vi "Data Viewer.vi"() -> ()   [LabVIEW 2014]
uses:
  TypeDef/Q1 Viewer.ctl
panel:
  out "ini file path":path
  out "Waveform Graph":waveform(dbl)[](graph)
  in  "Mode Selector":cluster{"Online Viewer":bool, "Navigator":bool}
  out "State":u16(ring) items=["initialize", "idle", "navigator", "online viewer", "exit"]
  in  "initialize":bool
  in  "referesh":bool
  in  "Cycle Time":i64=100 min=-1 step=1 format="%.0f msec"
  out "Sampling Interval":dbl min=0.0 step=1.0 format="%#_g msec"
  in  "Length (samples)":i64=1000 min=-1 step=1
  out "chart":waveform(dbl)[](graph)
  out "Start at sample":i32 min=0 step=1
  in  "Scrollbar":i32(c297)
  out "Number of Data":dbl format="%#_6f"
  in  "Variables":i32[](listbox)
  in  "Group Names":i32(listbox)
  in  "File Path Control":path caption="Open TDMS file:"
  out "Date":string
  out "Time":string
  in  "Stop Button":bool
  # "Data Viewer"
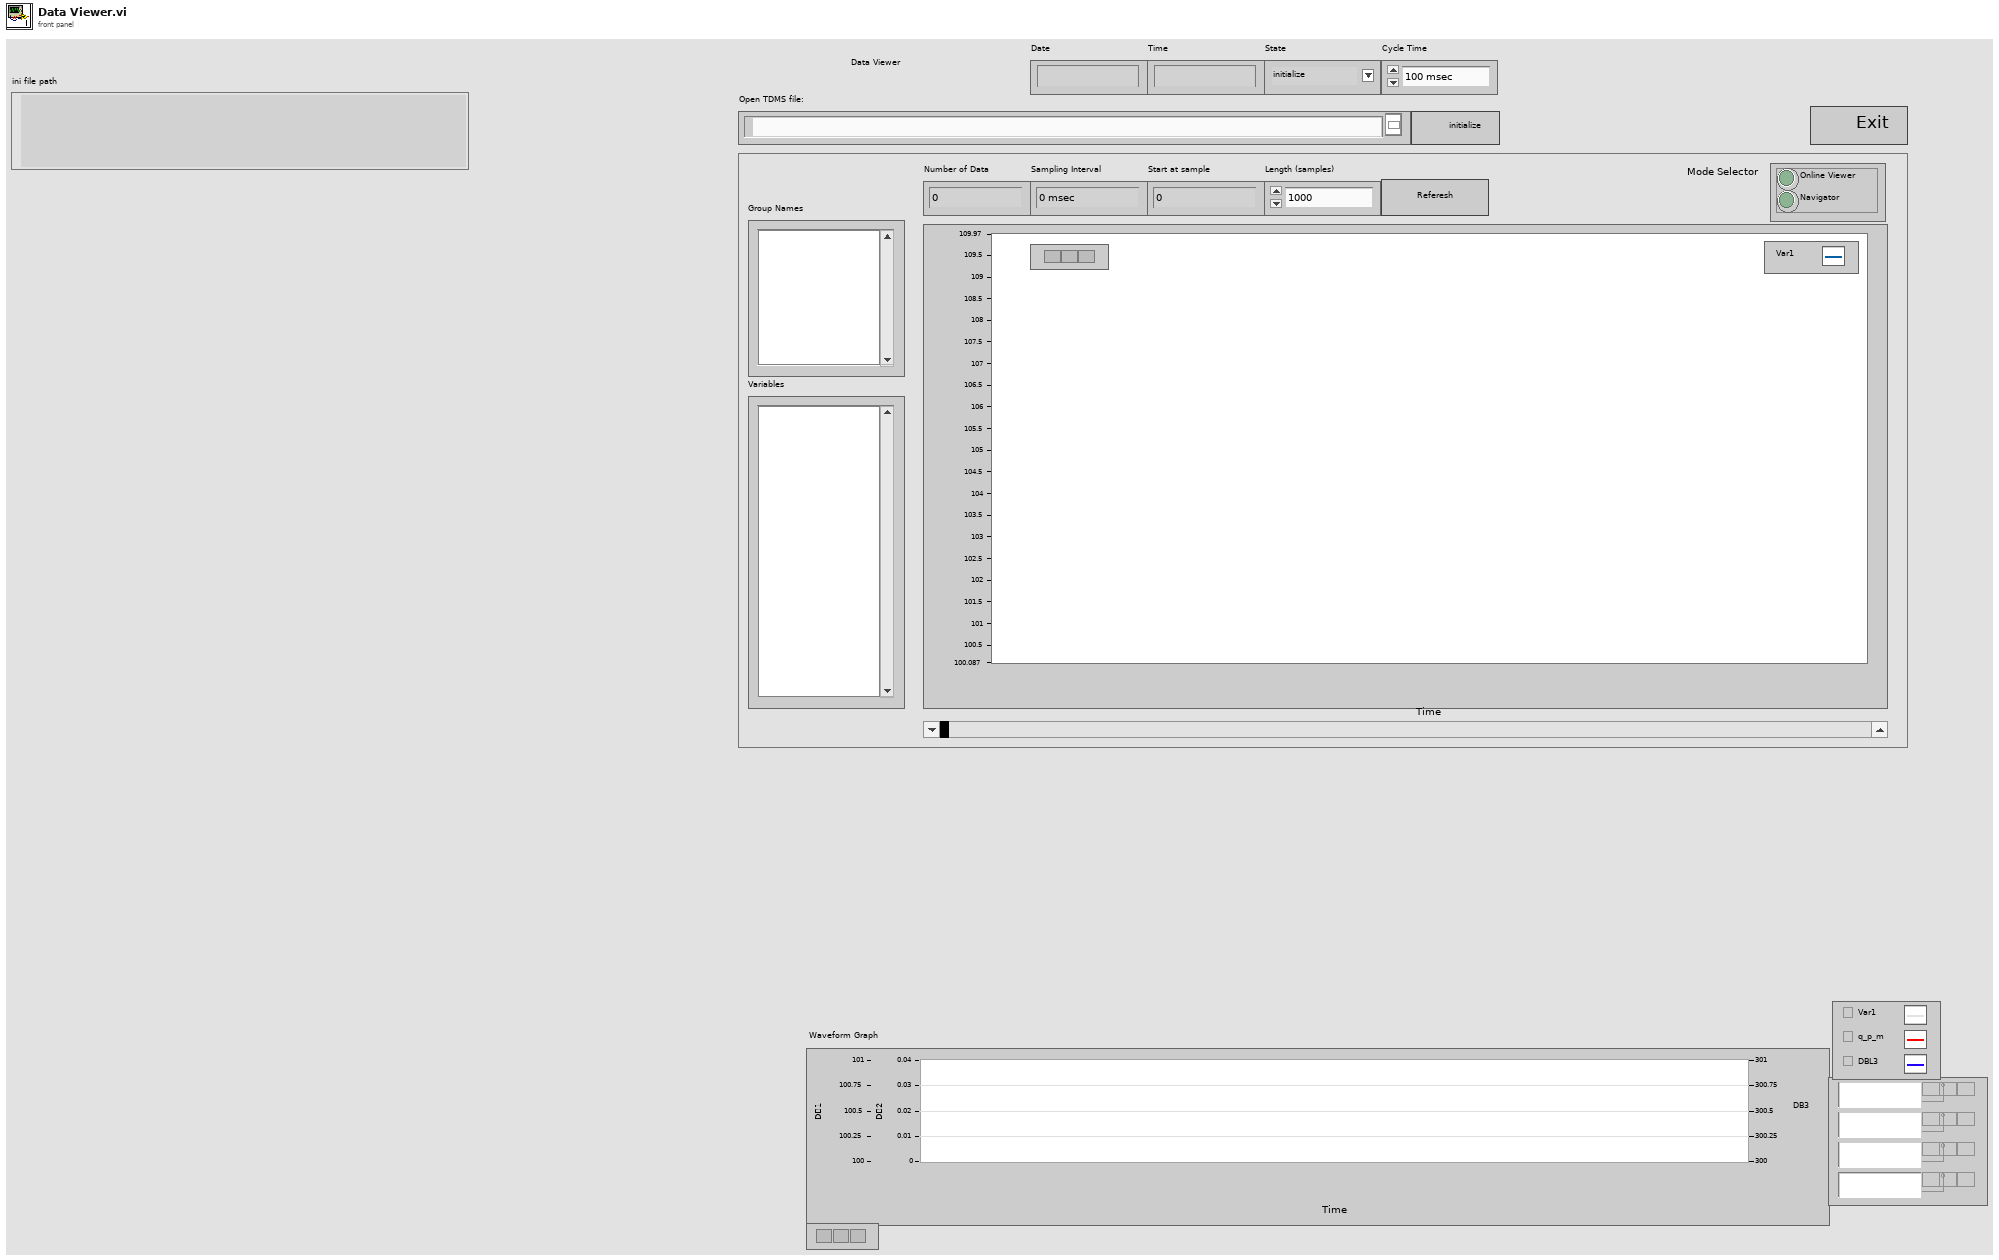
[diagram p1: front panel]
types:
  T1 = cluster{"Folder Path containing version information":path, "File name (including .ini)":path, "Section":string}
  T2 = typedef "Q1 Viewer.ctl" = cluster{"state":enum16{"initialize", "idle", "navigator", "online viewer", "exit"}, "data":variant}
  T3 = cluster{"path":path, "This VI":refnum<vi>, "Level of Application":u8}
  T4 = enum16{"open", "open or create", "create or replace", "create", "open (read-only)"}
  T5 = enum16{"initialize", "idle", "navigator", "online viewer", "exit"}
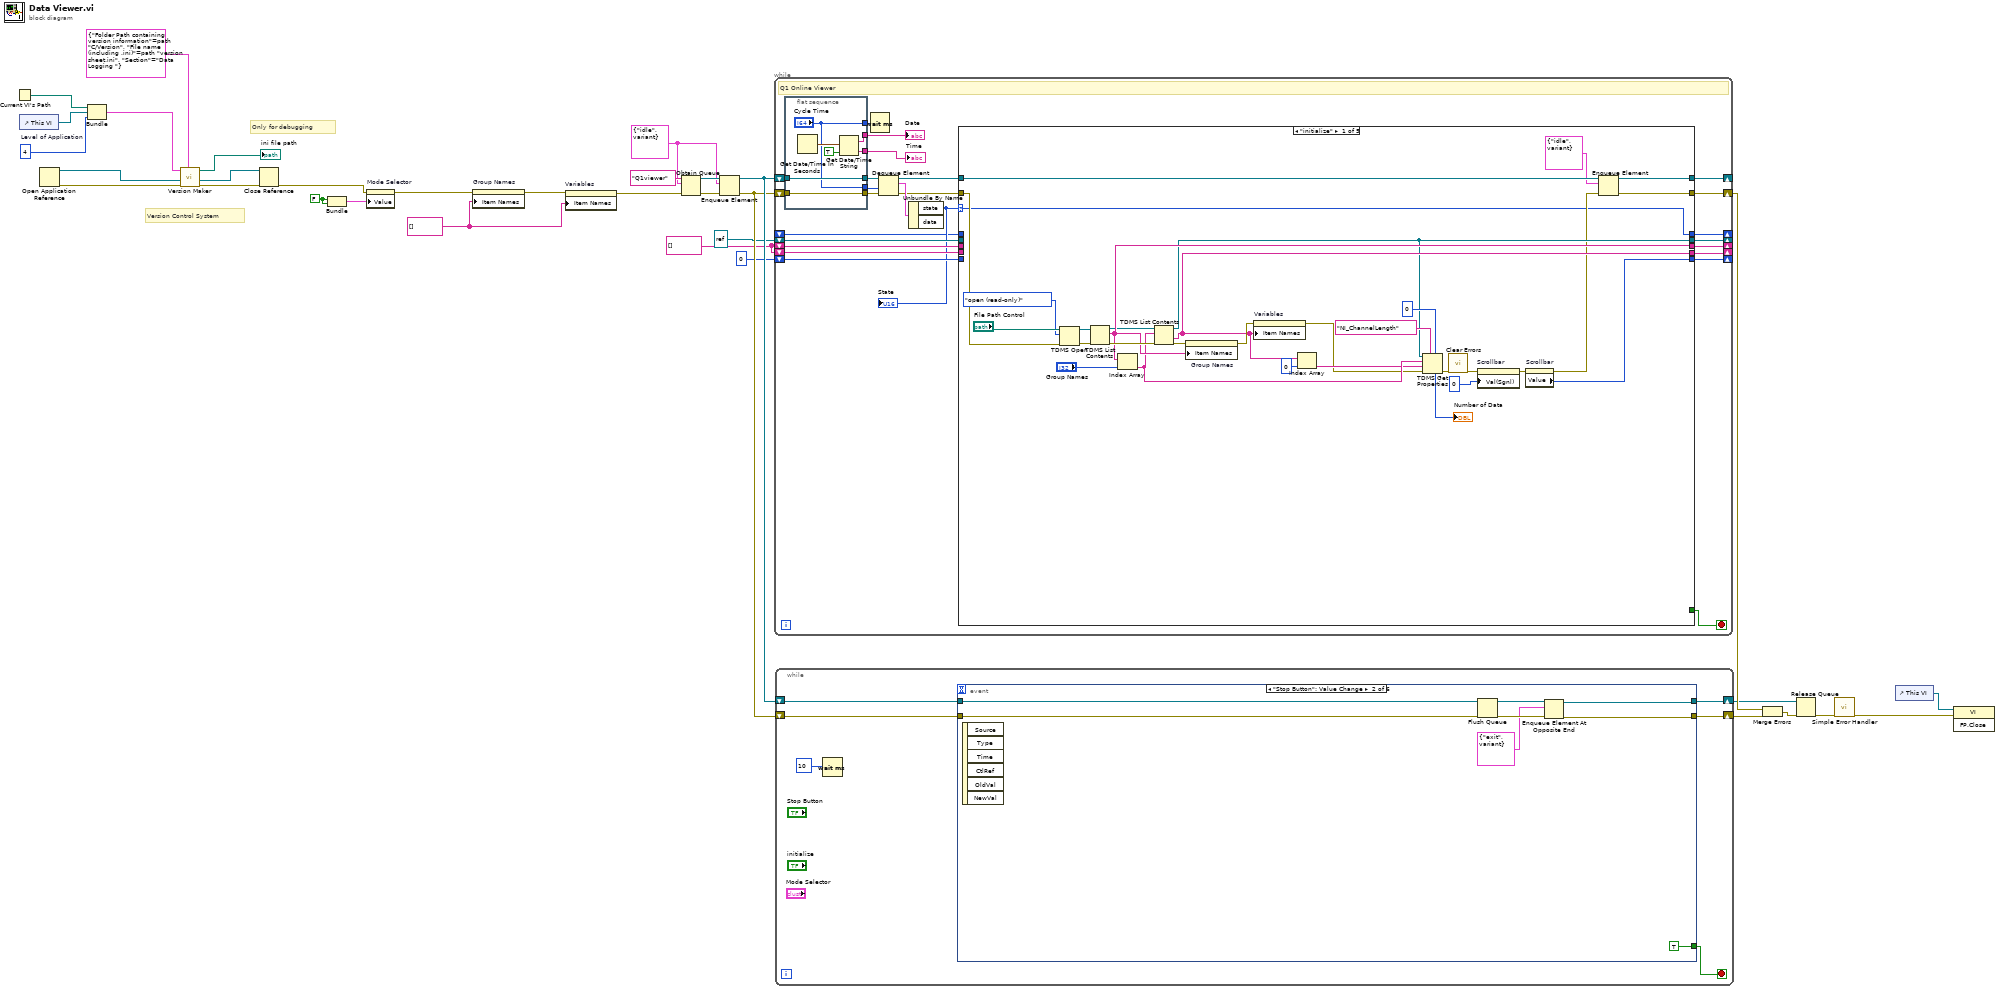
[diagram p0: block diagram]
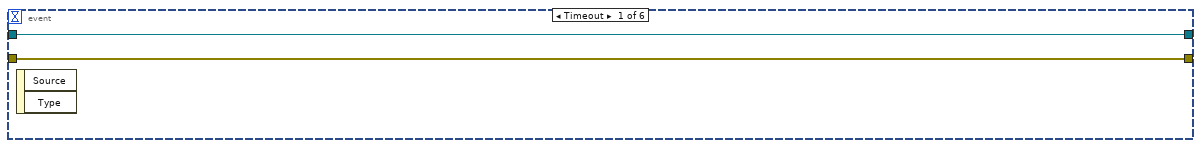
[diagram p2: hidden frame]
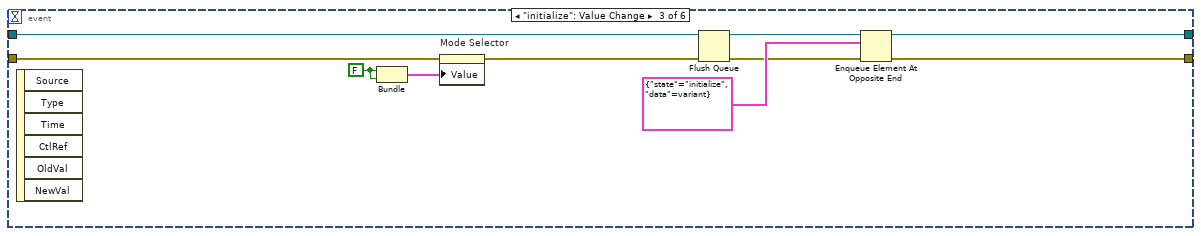
[diagram p3: hidden frame]
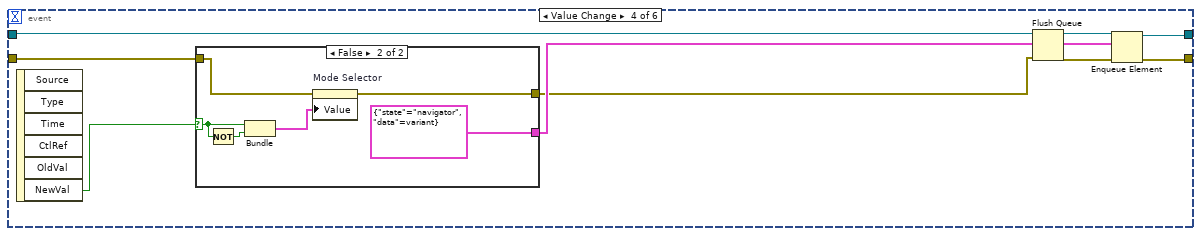
[diagram p4: hidden frame]
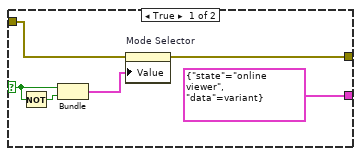
[diagram p5: hidden frame]
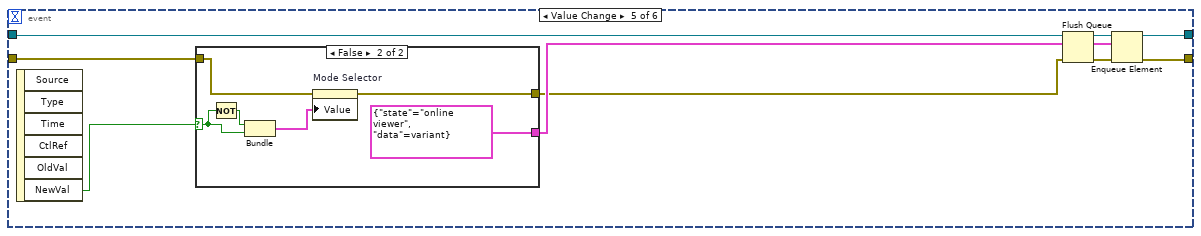
[diagram p6: hidden frame]
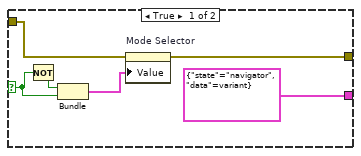
[diagram p7: hidden frame]
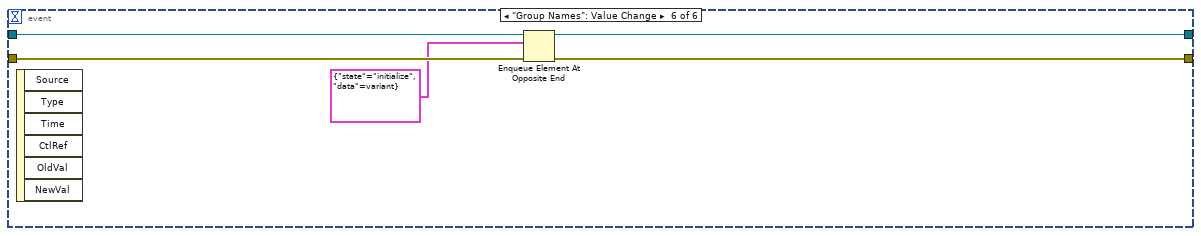
[diagram p8: hidden frame]
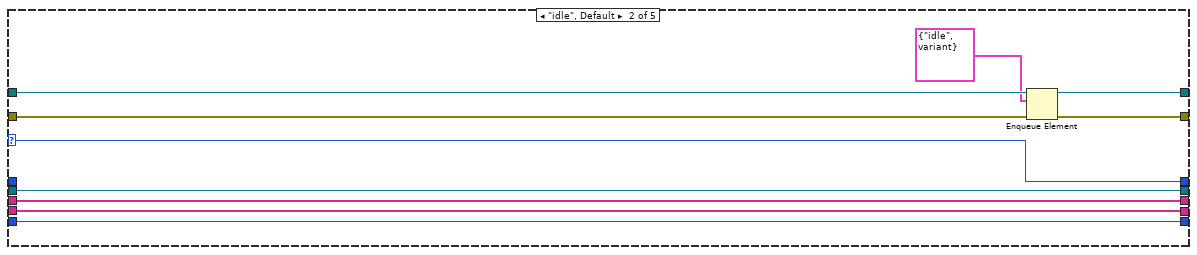
[diagram p9: hidden frame]
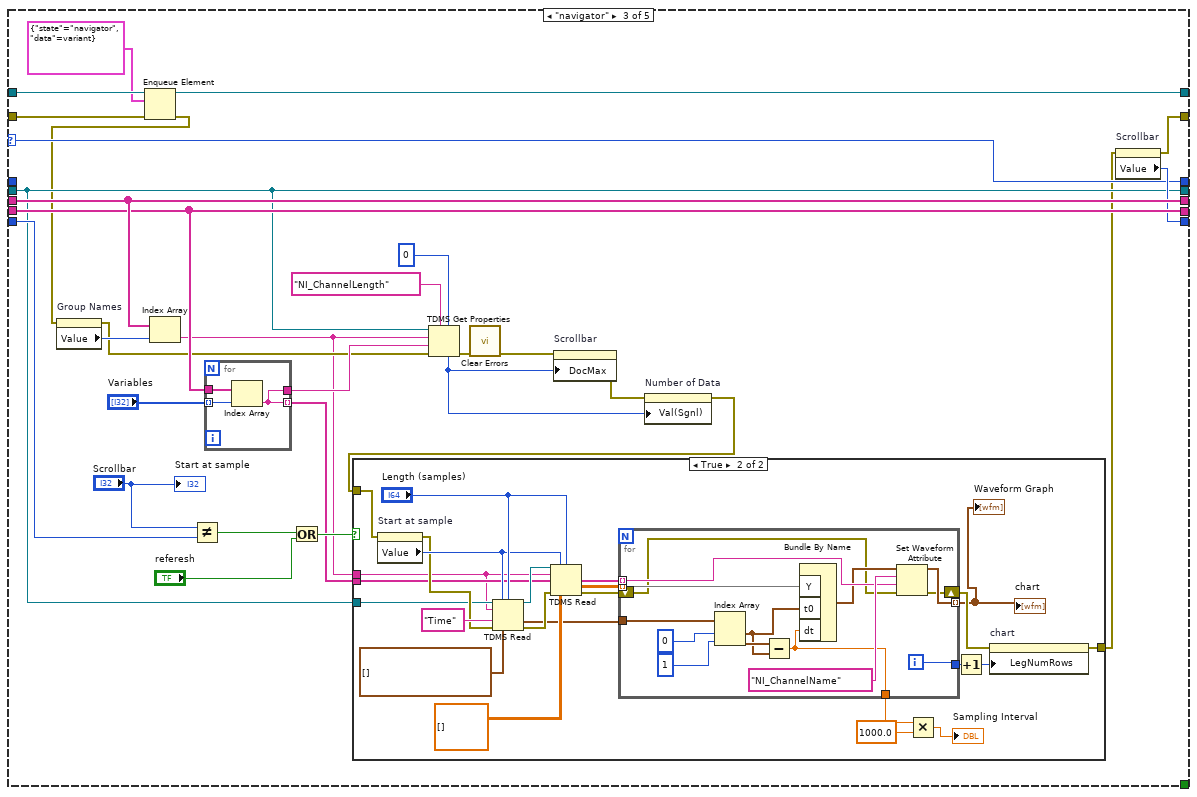
[diagram p10: hidden frame]
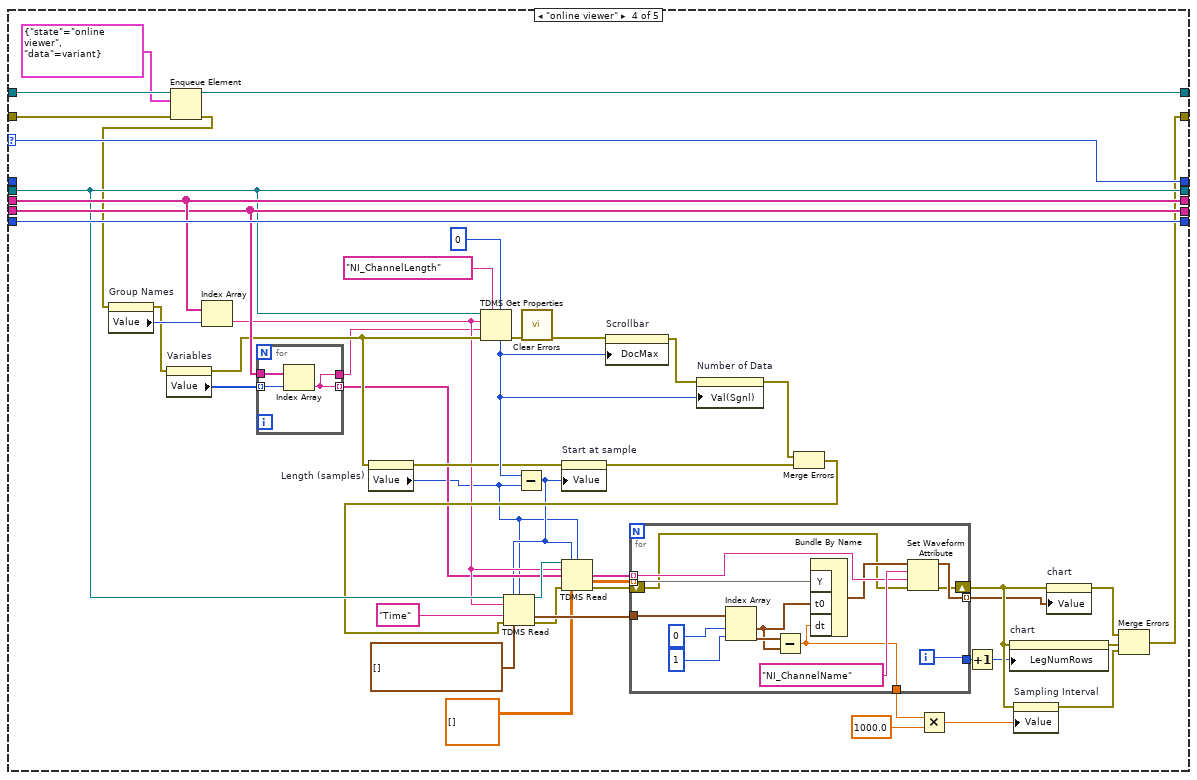
[diagram p12: hidden frame]
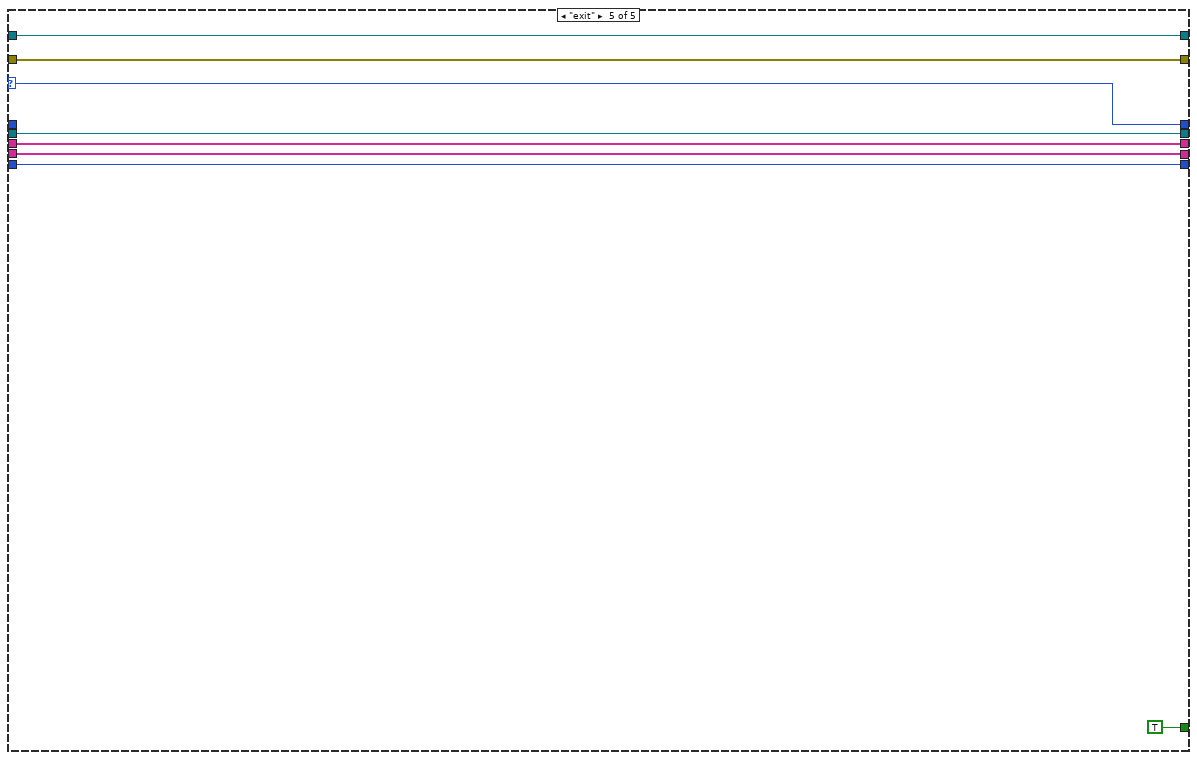
[diagram p13: hidden frame]
diagram:
  w6 = u8 4  # Level of Application
  w14 = FALSE
  w17 = string[] [] ("group names")
  w20 = T2 {"state"=enum."idle", "data"=variant}
  w22 = string[] [] ("group names")
  # "Only for debugging"
  # "Version Control System"
  n1 = Current VI's Path() -> (path=w4:path)
  n2 = control-ref of="This VI"() -> (w5:refnum<vi>)
  n3 = Open Application Reference() -> (0:w13:errorcluster, 3:w9:refnum<vi>)  [unwired: 4 in]
  n4 = Bundle("path"=w4, "This VI"=w5, "Level of Application"=w6) -> (w7:T3)  [unwired: 1 in]
  n5 = call "Version Maker.vi"("Version Sheet Cluster"=T1 {"Folder Path containing version information"=path "C:/Version", "File name (including .ini)"=path "version sheet.ini", "Section"="Data Logging "}, "Error In"=w13, "Open Application Reference in"=w9, "VI Information"=w7) -> ("Error Out"=w12:errorcluster, "Open Application Reference out"=w8:refnum<vi>, "Standard Config Path"=→"ini file path":path)  [unwired: 4 in, 1 out]
  n6 = Close Reference(reference=w8, error in (no error)=w12) -> (error out=w3:errorcluster)
  n7 = Bundle(w14, w14) -> (w15:cluster{bool, bool})  [unwired: 1 in]
  n8 = property on="Mode Selector" class="Clust (strict)"(error in=w3, "Value"=w15) -> (error out=w16:errorcluster)  [unwired: 1 in, 1 out]
  n9 = property on="Group Names" class="LstBox (strict)"(error in=w16, "Item Names"=w17) -> (error out=w19:errorcluster)  [unwired: 1 in, 1 out]
  n10 = property on="Variables" class="LstBox (strict)"(error in=w19, "Item Names"=w17) -> (error out=w18:errorcluster)  [unwired: 1 in, 1 out]
  n11 = Obtain Queue(name (unnamed)="Q1viewer", element data type=w20, error in (no error)=w18) -> (queue out=w32:refnum<queue>, error out=w31:errorcluster)  [unwired: 2 in, 1 out]
  n12 = Enqueue Element(queue=w32, element=w20, error in (no error)=w31) -> (queue out=w30:refnum<queue>, error out=w29:errorcluster)  [unwired: 1 in, 1 out]
  n13 = while {
    shift-right: [w53] -> _
    shift-left: w30 -> [w54]
    shift-right: [w52] -> w27
    shift-left: w29 -> [w58]
    shift-right: [w50] -> _
    shift-left: refnum<k34> refnum ("tdms file out") -> [w49]
    shift-right: [w48] -> _
    shift-left: w22 -> [w47]
    shift-right: [w46] -> _
    shift-left: w22 -> [w45]
    shift-right: [w44] -> _
    shift-left: 0 ("Scrollbar") -> [w43]
    shift-right: [w35] -> _
    shift-left: _ -> [w34]
    stop <- w51 stop-if-true
    # "Q1 Online Viewer"
    n14 = flat-sequence {
      tunnel: w58 -> [w247]
      tunnel: ["Cycle Time"] -> w57
      tunnel: [w250] -> w56
      tunnel: [w249] -> w55
      tunnel: w54 -> [w248]
      tunnel: [w248] -> w41
      tunnel: [w247] -> w39
      tunnel: ["Cycle Time"] -> w40
      frame #0 {
        n15 = Get Date/Time In Seconds() -> (seconds since 1Jan1904=w251:timestamp)
        n16 = Get Date/Time String(seconds (now)=w251, want seconds? (F)=TRUE) -> (date string=w250:string, time string=w249:string)  [unwired: 1 in]
      }
    }
    n17 = Wait (ms)(milliseconds to wait=w57) -> ()  [unwired: 1 out]
    n18 = Dequeue Element(queue=w41, timeout in ms (-1)=w40, error in (no error)=w39) -> (queue out=w37:refnum<queue>, element=w42:T2, error out=w38:errorcluster)  [unwired: 1 out]
    n19 = Unbundle By Name(w42) -> ("state"=w36:T5)  [unwired: 1 out]
    "State" <- w36
    n20 = case shown="\"initialize\"" w36 {
      selector: w36 -> [w59 w90 w103 w219 w238]
      tunnel: [w77 w93 w120 w207 w245] -> w53
      tunnel: w37 -> [w78 w94 w121 w209 w245]
      tunnel: [w76 w92 w113 w172 w244] -> w52
      tunnel: w38 -> [w87 w95 w101 w173 w244]
      tunnel: [_ _ _ _ TRUE] -> w51
      tunnel: [w70 w99 w111 w185 w242] -> w50
      tunnel: w49 -> [_ w99 w111 w185 w242]
      tunnel: [w81 w98 w126 w212 w241] -> w48
      tunnel: w47 -> [_ w98 w126 w212 w241]
      tunnel: [w74 w97 w124 w206 w240] -> w46
      tunnel: w45 -> [_ w97 w124 w206 w240]
      tunnel: [w63 w96 w114 w220 w239] -> w44
      tunnel: w43 -> [_ w96 w115 w220 w239]
      tunnel: [w59 w90 w103 w219 w238] -> w35
      tunnel: w34 -> [_ _ _ _ _]
      frame "initialize" {
        n21 = TDMS Open(8:w87, 10:T4."open (read-only)" ("operation (0:open)"), 11:"File Path Control") -> (0:w85:errorcluster, 3:w86:refnum<k34>)  [unwired: 4 in]
        n22 = TDMS List Contents(4:w85, 7:w86) -> (0:w83:errorcluster, 2:w81:string[], 3:w79:refnum<k34>)  [unwired: 1 in, 1 out]
        n23 = Index Array(array=w81, index="Group Names") -> (element=w69:string)
        n24 = TDMS List Contents(4:w83, 6:w69, 7:w79) -> (0:w82:errorcluster, 1:w74:string[], 3:w70:refnum<k34>)  [unwired: 1 out]
        n25 = property on="Group Names" class="LstBox (strict)"(error in=w82, "Item Names"=w81) -> (error out=w80:errorcluster)  [unwired: 1 in, 1 out]
        n26 = property on="Variables" class="LstBox (strict)"(error in=w80, "Item Names"=w74) -> (error out=w67:errorcluster)  [unwired: 1 in, 1 out]
        n27 = Index Array(array=w74, index=0) -> (element=w68:string)
        n28 = TDMS Get Properties(5:i64 0, 7:"NI_ChannelLength" ("channel name(s) in"), 8:w67, 9:w68, 10:w69, 11:w70) -> (0:w61:errorcluster, 4:→"Number of Data":i64)  [unwired: 4 out]
        n29 = call <vilib>:"Clear Errors.vi"("error in (no error)"=w61) -> ("error out"=w60:errorcluster)  [unwired: 5 in, 1 out]
        n30 = property on="Scrollbar" class="Scroll (strict)"(error in=w60, "Val(Sgnl)"=0 ("Value (Signaling)")) -> (error out=w64:errorcluster)  [unwired: 1 in, 1 out]
        n31 = property on="Scrollbar" class="Scroll (strict)"(error in=w64) -> (error out=w62:errorcluster, "Value"=w63:i32)  [unwired: 1 in, 1 out]
        n32 = Enqueue Element(queue=w78, element=T2 {"state"=enum."idle", "data"=variant}, error in (no error)=w62) -> (queue out=w77:refnum<queue>, error out=w76:errorcluster)  [unwired: 1 in, 1 out]
      }
      frame "idle", Default {
        n33 = Enqueue Element(queue=w94, element=T2 {"state"=enum."idle", "data"=variant}, error in (no error)=w95) -> (queue out=w93:refnum<queue>, error out=w92:errorcluster)  [unwired: 1 in, 1 out]
      }
      frame "navigator" {
        n34 = Enqueue Element(queue=w121, element=T2 {"state"=enum."navigator", "data"=variant}, error in (no error)=w101) -> (queue out=w120:refnum<queue>, error out=w100:errorcluster)  [unwired: 1 in, 1 out]
        n35 = property on="Group Names" class="LstBox (strict)"(error in=w100) -> (error out=w122:errorcluster, "Value"=w127:i32)  [unwired: 1 in, 1 out]
        n36 = Index Array(array=w126, index=w127) -> (element=w104:string)
        n37 = Not Equal?(x="Scrollbar", y=w115) -> (x != y?=w110:bool)
        n38 = for {
          tunnel: "Variables" -> [w171] mode=indexing
          tunnel: [w170] -> w105 mode=indexing
          tunnel: [w170] -> w123
          tunnel: w124 -> [w169]
          n39 = Index Array(array=w169, index=w171) -> (element=w170:string)
        }
        n40 = Or(x=w110, y="referesh") -> (x .or. y?=w108:bool)
        n41 = TDMS Get Properties(5:i64 0, 7:"NI_ChannelLength" ("channel name(s) in"), 8:w122, 9:w123, 10:w104, 11:w111) -> (0:w107:errorcluster, 4:w117:i64)  [unwired: 4 out]
        n42 = call <vilib>:"Clear Errors.vi"("error in (no error)"=w107) -> ("error out"=w106:errorcluster)  [unwired: 5 in, 1 out]
        n43 = property on="Scrollbar" class="Scroll (strict)"(error in=w106, "DocMax"=w117) -> (error out=w118:errorcluster)  [unwired: 1 in, 1 out]
        n44 = property on="Number of Data" class="DigNum (strict)"(error in=w118, "Val(Sgnl)"=w117) -> (error out=w116:errorcluster)  [unwired: 1 in, 1 out]
        n45 = case shown="True" w108 {
          tunnel: w116 -> [w130 w143]
          tunnel: [w130 w139] -> w102
          tunnel: w111 -> [_ w138]
          tunnel: w105 -> [_ w136]
          tunnel: w104 -> [_ w135]
          frame False {
          }
          frame True {
            n46 = property on="Start at sample" class="DigNum (strict)"(error in=w143) -> (error out=w142:errorcluster, "Value"=w144:i32)  [unwired: 1 in, 1 out]
            n47 = TDMS Read(0:w138, 1:w144, 2:"Length (samples)", 5:w135, 7:"Time", 11:w142, 12:timestamp[] []) -> (4:w137:refnum<k34>, 10:w148:timestamp[], 15:w151:errorcluster)  [unwired: 1 in, 3 out]
            n48 = TDMS Read(0:w137, 1:w144, 2:"Length (samples)", 5:w135, 7:w136, 11:w151, 12:dbl[][] []) -> (8:w147:string[], 10:w149:dbl[][], 15:w141:errorcluster)  [unwired: 1 in, 3 out]
            n49 = for {
              tunnel: w149 -> [w160] mode=indexing
              tunnel: w148 -> [w168]
              tunnel: [w158] -> w131 mode=indexing
              tunnel: w147 -> [w162] mode=indexing
              tunnel: [w161] -> w146
              shift-right: [w157] -> w140
              shift-left: w141 -> [w155]
              tunnel: [w156] -> w133
              i -> [w161]
              n50 = Index Array(array=w168, index #1=0 ("index"), index #2=1 ("index")) -> (element #1=w164:timestamp, element #2=w165:timestamp)
              n51 = Subtract(x=w165, y=w164) -> (x-y=w156:dbl)
              n52 = Bundle By Name("Y"=w160, "t0"=w164, "dt"=w156) -> (w159:waveform(dbl))  [unwired: 1 in]
              n53 = Set Waveform Attribute(4:w155, 5:w162, 6:"NI_ChannelName" ("name"), 7:w159) -> (0:w157:errorcluster, 3:w158:waveform(dbl))  [unwired: 1 out]
            }
            "chart" <- w131
            "Waveform Graph" <- w131
            n54 = Multiply(x=w133, y=1000.0) -> (x*y=→"Sampling Interval":dbl)
            n55 = Increment(x=w146) -> (x+1=w145:i32)
            n56 = property on="chart" class="WFChart (strict)"(error in=w140, "LegNumRows"=w145) -> (error out=w139:errorcluster)  [unwired: 1 in, 1 out]
          }
        }
        n57 = property on="Scrollbar" class="Scroll (strict)"(error in=w102) -> (error out=w113:errorcluster, "Value"=w114:i32)  [unwired: 1 in, 1 out]
        "Start at sample" <- "Scrollbar"
      }
      frame "online viewer" {
        n58 = Enqueue Element(queue=w209, element=T2 {"state"=enum."online viewer", "data"=variant}, error in (no error)=w173) -> (queue out=w207:refnum<queue>, error out=w174:errorcluster)  [unwired: 1 in, 1 out]
        n59 = property on="Group Names" class="LstBox (strict)"(error in=w174) -> (error out=w210:errorcluster, "Value"=w216:i32)  [unwired: 1 in, 1 out]
        n60 = property on="Variables" class="LstBox (strict)"(error in=w210) -> (error out=w184:errorcluster, "Value"=w211:i32[])  [unwired: 1 in, 1 out]
        n61 = Index Array(array=w212, index=w216) -> (element=w179:string)
        n62 = for {
          tunnel: w211 -> [w237] mode=indexing
          tunnel: [w236] -> w177 mode=indexing
          tunnel: [w236] -> w178
          tunnel: w206 -> [w235]
          n63 = Index Array(array=w235, index=w237) -> (element=w236:string)
        }
        n64 = property on="Length (samples)" class="DigNum (strict)"(error in=w184) -> (error out=w183:errorcluster, "Value"=w175:i64)  [unwired: 1 in, 1 out]
        n65 = TDMS Get Properties(5:i64 0, 7:"NI_ChannelLength" ("channel name(s) in"), 8:w184, 9:w178, 10:w179, 11:w185) -> (0:w214:errorcluster, 4:w205:i64)  [unwired: 4 out]
        n66 = Subtract(x=w205, y=w175) -> (x-y=w176:i64)
        n67 = call <vilib>:"Clear Errors.vi"("error in (no error)"=w214) -> ("error out"=w213:errorcluster)  [unwired: 5 in, 1 out]
        n68 = property on="Start at sample" class="DigNum (strict)"(error in=w183, "Value"=w176) -> (error out=w181:errorcluster)  [unwired: 1 in, 1 out]
        n69 = property on="Scrollbar" class="Scroll (strict)"(error in=w213, "DocMax"=w205) -> (error out=w215:errorcluster)  [unwired: 1 in, 1 out]
        n70 = property on="Number of Data" class="DigNum (strict)"(error in=w215, "Val(Sgnl)"=w205) -> (error out=w182:errorcluster)  [unwired: 1 in, 1 out]
        n71 = Merge Errors(w182, w181) -> (w180:errorcluster)
        n72 = TDMS Read(0:w185, 1:w176, 2:w175, 5:w179, 7:"Time", 11:w180, 12:timestamp[] []) -> (4:w195:refnum<k34>, 10:w191:timestamp[], 15:w188:errorcluster)  [unwired: 1 in, 3 out]
        n73 = TDMS Read(0:w195, 1:w176, 2:w175, 5:w179, 7:w177, 11:w188, 12:dbl[][] []) -> (8:w192:string[], 10:w190:dbl[][], 15:w194:errorcluster)  [unwired: 1 in, 3 out]
        n74 = for {
          tunnel: w190 -> [w226] mode=indexing
          tunnel: w191 -> [w234]
          tunnel: [w224] -> w198 mode=indexing
          tunnel: w192 -> [w228] mode=indexing
          tunnel: [w227] -> w193
          shift-right: [w223] -> w203
          shift-left: w194 -> [w221]
          tunnel: [w222] -> w196
          i -> [w227]
          n75 = Index Array(array=w234, index #1=0 ("index"), index #2=1 ("index")) -> (element #1=w230:timestamp, element #2=w231:timestamp)
          n76 = Subtract(x=w231, y=w230) -> (x-y=w222:dbl)
          n77 = Bundle By Name("Y"=w226, "t0"=w230, "dt"=w222) -> (w225:waveform(dbl))  [unwired: 1 in]
          n78 = Set Waveform Attribute(4:w221, 5:w228, 6:"NI_ChannelName" ("name"), 7:w225) -> (0:w223:errorcluster, 3:w224:waveform(dbl))  [unwired: 1 out]
        }
        n79 = Multiply(x=w196, y=1000.0) -> (x*y=w202:dbl)
        n80 = Increment(x=w193) -> (x+1=w199:i32)
        n81 = property on="chart" class="WFChart (strict)"(error in=w203, "LegNumRows"=w199) -> (error out=w200:errorcluster)  [unwired: 1 in, 1 out]
        n82 = property on="Sampling Interval" class="DigNum (strict)"(error in=w203, "Value"=w202) -> (error out=w204:errorcluster)  [unwired: 1 in, 1 out]
        n83 = property on="chart" class="WFChart (strict)"(error in=w203, "Value"=w198) -> (error out=w201:errorcluster)  [unwired: 1 in, 1 out]
        n84 = Merge Errors(w201, w200, w204) -> (w172:errorcluster)
      }
      frame "exit" {
      }
    }
    "Time" <- w55
    "Date" <- w56
  }
  n85 = while {
    shift-right: [w256] -> w26
    shift-left: w30 -> [w258]
    shift-right: [w255] -> w28
    shift-left: w29 -> [w257]
    stop <- w254 stop-if-true
    n86 = Wait (ms)(milliseconds to wait=u32 10) -> ()  [unwired: 1 out]
    n87 = event shown="[1] \"Stop Button\": Value Change" {
      selector: _ -> [_ _ _ _ _ _]
      dyn-events: _ -> [_ _ _ _ _ _]
      timeout: _ -> [_ _ _ _ _ _]
      tunnel: w258 -> [w260 w267 w270 w281 w301 w325]
      tunnel: w257 -> [w259 w266 w269 w280 w300 w324]
      tunnel: [w260 w262 w278 w287 w308 w323] -> w256
      tunnel: [w259 w263 w276 w286 w307 w322] -> w255
      tunnel: [_ TRUE _ _ _ _] -> w254
      event Timeout {
        n88 = event-data() -> ()  [unwired: 1 in, 2 out]
      }
      event "Stop Button": Value Change {
        n89 = event-data() -> ()  [unwired: 1 in, 6 out]
        n90 = Flush Queue(queue=w267, error in (no error)=w266) -> (queue out=w265:refnum<queue>, error out=w264:errorcluster)  [unwired: 1 out]
        n91 = Enqueue Element At Opposite End(queue=w265, element=T2 {"state"=enum."exit", "data"=variant}, error in (no error)=w264) -> (queue out=w262:refnum<queue>, error out=w263:errorcluster)  [unwired: 1 in, 1 out]
      }
      event "initialize": Value Change {
        w273 = FALSE
        n92 = event-data() -> ()  [unwired: 1 in, 6 out]
        n93 = Bundle(w273, w273) -> (w274:cluster{bool, bool})  [unwired: 1 in]
        n94 = property on="Mode Selector" class="Clust (strict)"(error in=w269, "Value"=w274) -> (error out=w271:errorcluster)  [unwired: 1 in, 1 out]
        n95 = Flush Queue(queue=w270, error in (no error)=w271) -> (queue out=w275:refnum<queue>, error out=w272:errorcluster)  [unwired: 1 out]
        n96 = Enqueue Element At Opposite End(queue=w275, element=T2 {"state"=enum."initialize", "data"=variant}, error in (no error)=w272) -> (queue out=w278:refnum<queue>, error out=w276:errorcluster)  [unwired: 1 in, 1 out]
      }
      event "Mode Selector.Online Viewer": Value Change {
        n97 = event-data() -> ("NewVal"=w285:bool)  [unwired: 1 in, 5 out]
        n98 = case shown="False" w285 {
          selector: w285 -> [w292 w298]
          tunnel: w280 -> [w291 w297]
          tunnel: [w289 w295] -> w282
          tunnel: [T2 {"state"=enum."online viewer", "data"=variant} T2 {"state"=enum."navigator", "data"=variant}] -> w284
          frame True {
            n99 = Not(x=w292) -> (.not. x?=w293:bool)
            n100 = Bundle(w292, w293) -> (w290:cluster{bool, bool})  [unwired: 1 in]
            n101 = property on="Mode Selector" class="Clust (strict)"(error in=w291, "Value"=w290) -> (error out=w289:errorcluster)  [unwired: 1 in, 1 out]
          }
          frame False {
            n102 = Not(x=w298) -> (.not. x?=w299:bool)
            n103 = Bundle(w298, w299) -> (w296:cluster{bool, bool})  [unwired: 1 in]
            n104 = property on="Mode Selector" class="Clust (strict)"(error in=w297, "Value"=w296) -> (error out=w295:errorcluster)  [unwired: 1 in, 1 out]
          }
        }
        n105 = Flush Queue(queue=w281, error in (no error)=w282) -> (queue out=w279:refnum<queue>, error out=w283:errorcluster)  [unwired: 1 out]
        n106 = Enqueue Element(queue=w279, element=w284, error in (no error)=w283) -> (queue out=w287:refnum<queue>, error out=w286:errorcluster)  [unwired: 1 in, 1 out]
      }
      event "Mode Selector.Navigator": Value Change {
        n107 = event-data() -> ("NewVal"=w305:bool)  [unwired: 1 in, 5 out]
        n108 = case shown="False" w305 {
          selector: w305 -> [w310 w315]
          tunnel: w300 -> [w314 w320]
          tunnel: [w312 w318] -> w302
          tunnel: [T2 {"state"=enum."navigator", "data"=variant} T2 {"state"=enum."online viewer", "data"=variant}] -> w304
          frame True {
            n109 = Not(x=w310) -> (.not. x?=w309:bool)
            n110 = Bundle(w309, w310) -> (w313:cluster{bool, bool})  [unwired: 1 in]
            n111 = property on="Mode Selector" class="Clust (strict)"(error in=w314, "Value"=w313) -> (error out=w312:errorcluster)  [unwired: 1 in, 1 out]
          }
          frame False {
            n112 = Not(x=w315) -> (.not. x?=w316:bool)
            n113 = Bundle(w316, w315) -> (w319:cluster{bool, bool})  [unwired: 1 in]
            n114 = property on="Mode Selector" class="Clust (strict)"(error in=w320, "Value"=w319) -> (error out=w318:errorcluster)  [unwired: 1 in, 1 out]
          }
        }
        n115 = Flush Queue(queue=w301, error in (no error)=w302) -> (queue out=w306:refnum<queue>, error out=w303:errorcluster)  [unwired: 1 out]
        n116 = Enqueue Element(queue=w306, element=w304, error in (no error)=w303) -> (queue out=w308:refnum<queue>, error out=w307:errorcluster)  [unwired: 1 in, 1 out]
      }
      event "Group Names": Value Change {
        n117 = event-data() -> ()  [unwired: 1 in, 6 out]
        n118 = Enqueue Element At Opposite End(queue=w325, element=T2 {"state"=enum."initialize", "data"=variant}, error in (no error)=w324) -> (queue out=w323:refnum<queue>, error out=w322:errorcluster)  [unwired: 1 in, 1 out]
      }
    }
  }
  n119 = Merge Errors(w27, w28) -> (w25:errorcluster)
  n120 = Release Queue(queue=w26, error in (no error)=w25) -> (error out=w24:errorcluster)  [unwired: 1 in, 2 out]
  n121 = call <vilib>:"Simple Error Handler.vi"("error in (no error)"=w24) -> ("error out"=w1:errorcluster)  [unwired: 4 in, 4 out]
  n122 = control-ref of="This VI"() -> (w2:refnum<vi>)
  n123 = invoke class="VI" method="FP.Close"(reference=w2, error in=w1) -> ()  [unwired: 1 in, 3 out]
